vi "Default Broadcast--template.vi"(8 "error in (no error)":errorcluster) -> (0 "error out":errorcluster, 1 "Update Module Execution Status":refnum<user-event>, 2 "Error Reported":refnum<user-event>, 3 "Status Updated":refnum<user-event>, 4 "System Message":refnum<user-event>, 5 "Module Did Stop":refnum<user-event>)   [LabVIEW 2014, in "hse-dqmh-dynamicrequesters.lvlib"]
doc: "____\nHAMPEL SOFTWARE ENGINEERING v0.7.0 (2018-07-16 18:12)"
uses:
  hse-dqmh-dynamicrequesters.lvlib
  Stop Argument--cluster.ctl
  Status Updated Argument--cluster.ctl
  Error Reported Argument--cluster.ctl
  Get Module Execution Status Argument--cluster.ctl
  Controls/System Message Argument--cluster.ctl
  Controls/System Message Source.ctl
  hse-dqmh.lvlib
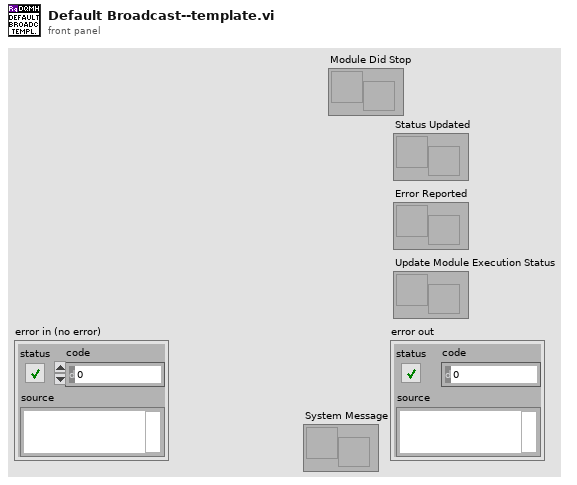
[diagram p1: front panel]
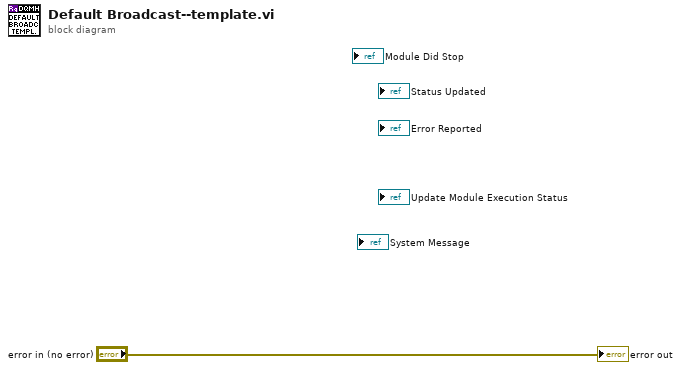
[diagram p0: block diagram]
diagram:
  "error out" <- "error in (no error)"
